vi "Calculate Amplitude at Target Frequency.vi"(7 "Target frequency":dbl, 10 "Amplitudes":dbl[](array[numeric]), 11 "Frequencies":dbl[](array[numeric])) -> (1 "Amplitude @ target frequency":dbl)   [LabVIEW 2021, in "audio_adc_frequencyResponseMeasurement.lvlib"]
uses:
  audio_adc_frequencyResponseMeasurement.lvlib
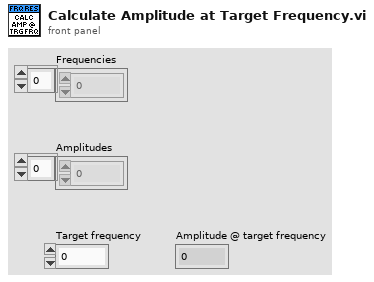
[diagram p1: front panel]
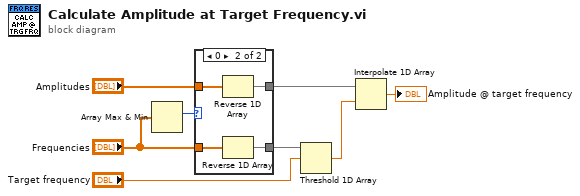
[diagram p0: block diagram]
diagram:
  n1 = Array Max & Min(array="Frequencies") -> (max index (indices)=w1:i32)  [unwired: 3 out]
  n2 = case shown="0" w1 {
    tunnel: "Frequencies" -> [w10 w14]
    tunnel: [w10 w13] -> w6
    tunnel: "Amplitudes" -> [w9 w12]
    tunnel: [w9 w11] -> w4
    frame Default {
    }
    frame 0 {
      n3 = Reverse 1D Array(array=w12) -> (reversed array=w11:dbl[])
      n4 = Reverse 1D Array(array=w14) -> (reversed array=w13:dbl[])
    }
  }
  n5 = Threshold 1D Array(2:"Target frequency", 3:w6) -> (0:w3:dbl)  [unwired: 1 in]
  n6 = Interpolate 1D Array(1:w3, 2:w4) -> (0:→"Amplitude @ target frequency":dbl)
